vi "comp_stop.vi"(0 "VISA resource name":refnum<visa-resource-name>, 1 "Relax Time":i32 min=-1000000 max=1000000, 5 "Master Axis":i32, 7 "Slave Axis":i32, 11 "error in (no error)":errorcluster, 12 "relax":dbl format="%.6f") -> (4 "VISA resource name out":refnum<visa-resource-name>, 15 "error out":errorcluster)   [LabVIEW 2009]
uses:
  <instrlib>/Newport ESP301/Newport ESP301.lvlib
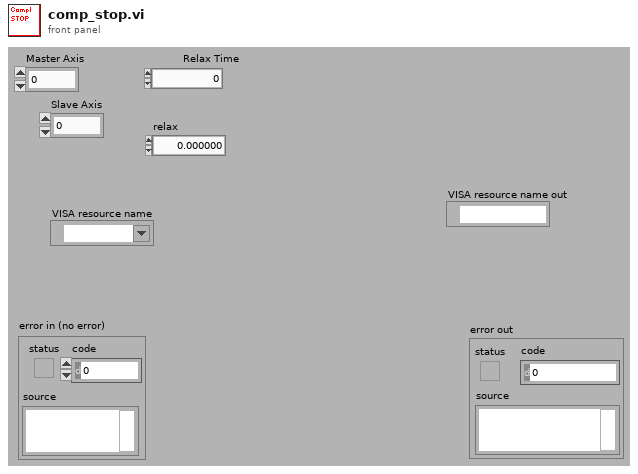
[diagram p1: front panel]
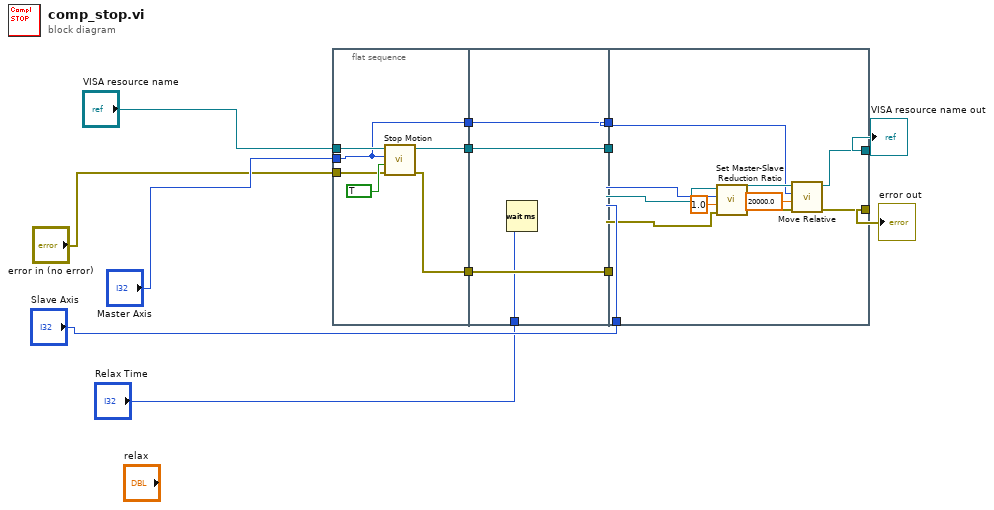
[diagram p0: block diagram]
diagram:
  n1 = flat-sequence {
    tunnel: "VISA resource name" -> [w18]
    tunnel: "Master Axis" -> [w14]
    tunnel: "error in (no error)" -> [w17]
    tunnel: [w16] -> w7
    tunnel: [w15] -> w5
    tunnel: [w14] -> w3
    tunnel: w7 -> [w23]
    tunnel: [w23] -> w6
    tunnel: w5 -> [w22]
    tunnel: [w22] -> w4
    tunnel: w3 -> [w21]
    tunnel: [w21] -> w2
    tunnel: "Relax Time" -> [w20]
    tunnel: w6 -> [w24]
    tunnel: w4 -> [w25]
    tunnel: w2 -> [w30]
    tunnel: "Slave Axis" -> [w33]
    tunnel: [w27] -> w9
    tunnel: [w26] -> w8
    frame #0 {
      n2 = call <instrlib>:"Stop Motion.vi"("error in (no error)"=w17, "Stop all axes (F)"=TRUE, "Axis (1)"=w14, "VISA resource name"=w18) -> ("error out"=w16:errorcluster, "VISA resource name out"=w15:refnum<visa-resource-name>)  [unwired: 2 in]
    }
    frame #1 {
      n3 = Wait (ms)(milliseconds to wait=w20) -> ()  [unwired: 1 out]
    }
    frame #2 {
      n4 = call <instrlib>:"Set Master-Slave Reduction Ratio.vi"("error in (no error)"=w24, "Reduction Ratio (0)"=1.0, "Axis (1)"=w33, "VISA resource name"=w25) -> ("error out"=w29:errorcluster, "VISA resource name out"=w31:refnum<visa-resource-name>)  [unwired: 2 in]
      n5 = call <instrlib>:"Move Relative.vi"("error in (no error)"=w29, "Position (0 units)"=20000.0, "Axis (1)"=w30, "VISA resource name"=w31) -> ("error out"=w27:errorcluster, "VISA resource name out"=w26:refnum<visa-resource-name>)  [unwired: 2 in]
    }
  }
  "error out" <- w9
  "VISA resource name out" <- w8
